vi "TRAJECTORY_CREATE_CUBIC_BEGIN.vi"() -> (0 "Trajectory \ncalculation \nerror":errorcluster, 2 "Trajectory Items":i32, 3 "TotalTImeSecs":dbl)   [LabVIEW 2019]
uses:
  <vilib>/Rock Robotics/WPI/ThirdParty/JAS_Junk/TrajLib/Rotation_CreateAngle.vi
  <vilib>/Rock Robotics/WPI/ThirdParty/JAS_Junk/TrajLib/DiffDriveKinematicsConstraint_New.vi
  <vilib>/Rock Robotics/WPI/ThirdParty/JAS_Junk/TrajLib/CentripetalAccelConstraint_New.vi
  <vilib>/Rock Robotics/WPI/ThirdParty/JAS_Junk/TrajLib/Trajectory_Library.lvlib
panel:
  in  "Interior WayPoints":cluster{"X Inches":dbl, "Y Inches":dbl}[](array[cluster])=[{"X Inches"=105.0, "Y Inches"=65.0}]
  in  "Output Position":T1={"X Inches"=210.0, "Y Inches"=106.0, "Heading\nDegrees"=45.0}
  in  "Input Position":T1={"X Inches"=15.0, "Y Inches"=105.0, "Heading\nDegrees"=-45.0}
  in  "Use Diff Drive\nKinematic\nConstraint":bool=TRUE
  in  "Use Centripetal\nAcceleration\nConstaint":bool=TRUE
  out "Wheelbase Width":dbl=0.66 format="%20.4f"
  out "MaxAcceleration":dbl=1.3 format="%17.4f"
  out "MaxVelocity":dbl=2.0 format="%17.4f"
  out "Max Cent Accel":dbl=1.0 format="%20.4f"
  in  "Max Cent Accel INCHES/SEC^2":dbl=15.0 format="%20.1f"
  in  "Wheelbase Width INCHES":dbl=50.0 format="%20.1f"
  in  "MaxAcceleration INCHES/SEC^2":dbl=35.0 format="%17.1f"
  in  "MaxVelocity  INCHES/SEC":dbl=45.0 format="%17.1f"
  # "TRAJECTORY CONFIGURATION"
  # "real 20.9"
  # "TRAJECTORY DEFINITION"
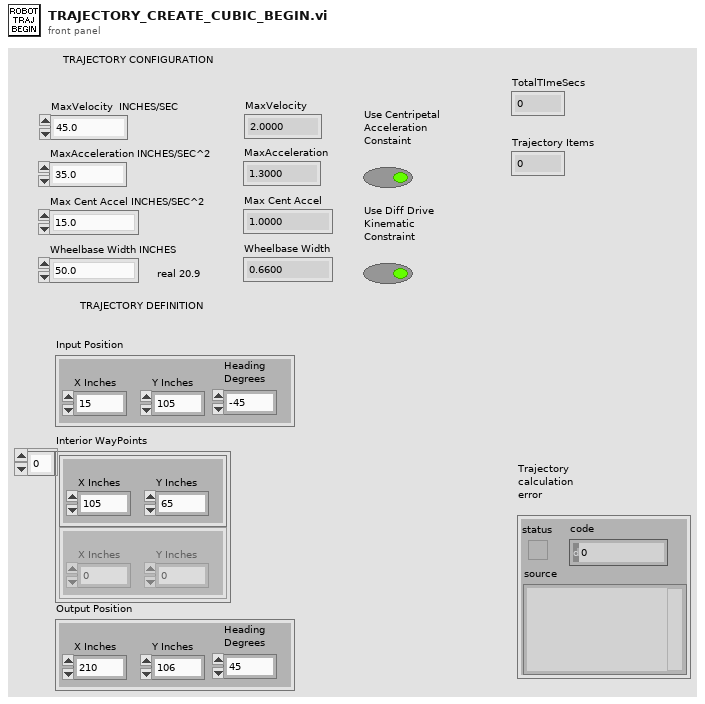
[diagram p1: front panel]
types:
  T1 = cluster{"X Inches":dbl, "Y Inches":dbl, "Heading\nDegrees":dbl}
  T2 = typedef "Trajectory_Library.lvlib/TRANSLATION2D.ctl" = cluster{"X":dbl, "Y":dbl}
  T3 = typedef "Trajectory_Library.lvlib/POSE2D.ctl" = cluster{"TRANSLATION":T2, "ROTATION":T4}
  T4 = typedef "Trajectory_Library.lvlib/ROTATION2D.ctl" = cluster{"VALUE":dbl, "COS":dbl, "SIN":dbl}
  T5 = typedef "Trajectory_Library.lvlib/TRAJ_CONFIG.ctl" = cluster{"MaxVelocity":dbl, "Max Acceleration":dbl, "StartVelocity":dbl, "End Velocity":dbl, "Reversed":bool, "DiffDrKineConstntDefined":bool, "CentAcellConstntDefined":bool, "DiffDrVoltConstntDefined":bool, "DIFF_DRIVE_KINE_CONSTRAINT":T6, "CENTRIPETAL_ACCEL_CONSTRAINT":T8, "SwerveDrKineConstntDefined":bool, "SWERVE_DRIVE_KINE_CONSTRAINT":T9, "DIFF_DRIVE_VOLTAGE_CONSTRAINT":T12, "MECANUM_DRIVE_KINE_CONSTRAINT":T14, "MecanumDrKineConstntDefined":bool}
  T6 = typedef "Trajectory_Library.lvlib/TRAJ_CONSTRAINT_DIIF_DRIVE_KINEMATICS.ctl" = cluster{"Max Speed (M/S)":dbl, "DIFF_DRIVE_KINEMATICS":T7}
  T7 = typedef "Trajectory_Library.lvlib/DIFF_DRIVE_KINEMATICS.ctl" = cluster{"TrackWidth_Meters":dbl}
  T8 = typedef "Trajectory_Library.lvlib/TRAJ_CONSTRAINT_CENTRIPETAL_ACCEL.ctl" = cluster{"Max Cent Accel":dbl}
  T9 = typedef "Trajectory_Library.lvlib/TRAJ_CONSTRAINT_SWERVE_DRIVE_KINEMATICS.ctl" = cluster{"Max Speed (M/S)":dbl, "SwerveKinematics":T10}
  T10 = typedef "Trajectory_Library.lvlib/SWERVE_DRIVE_KINEMATICS.ctl" = cluster{"NumModules":i32, "InverseKinematics":T11, "ForwardKinematics":T11, "Modules":T2[], "PrevCoR":T2}
  T11 = typedef "NI_Matrix.lvlib/RealMatrix.ctl" = dbl[][]
  T12 = typedef "Trajectory_Library.lvlib/TRAJ_CONSTRAINT_DIIF_DRIVE_VOLTAGE.ctl" = cluster{"Max Voltage":dbl, "DIFF_DRIVE_KINEMATICS":T7, "SIMPLE_MOTOR_FF":T13}
  T13 = typedef "Trajectory_Library.lvlib/SIMPLE_MOTOR_FF.ctl" = cluster{"Ks":dbl, "Kv":dbl, "Ka":dbl}
  T14 = typedef "Trajectory_Library.lvlib/TRAJ_CONSTRAINT_MECA_DRIVE_KINEMATICS.ctl" = cluster{"Max Speed (M/S)":dbl, "MECA_DRIVE_KINEMATICS":T15}
  T15 = typedef "Trajectory_Library.lvlib/MECA_DRIVE_KINEMATICS.ctl" = cluster{"FrontLeft":T2, "FrontRight":T2, "RearLeft":T2, "RearRight":T2, "InverseKinematics":T11, "ForwardKinematics":T11, "PrevCoR":T2}
  T16 = typedef "Trajectory_Library.lvlib/TRAJECTORY.ctl" = cluster{"TotalTImeSecs":dbl, "States":T17[]}
  T17 = typedef "Trajectory_Library.lvlib/TRAJ_STATE.ctl" = cluster{"TimeSeconds":dbl, "Velocity":dbl, "Acceleration":dbl, "POSE":T3, "Curvature":dbl}
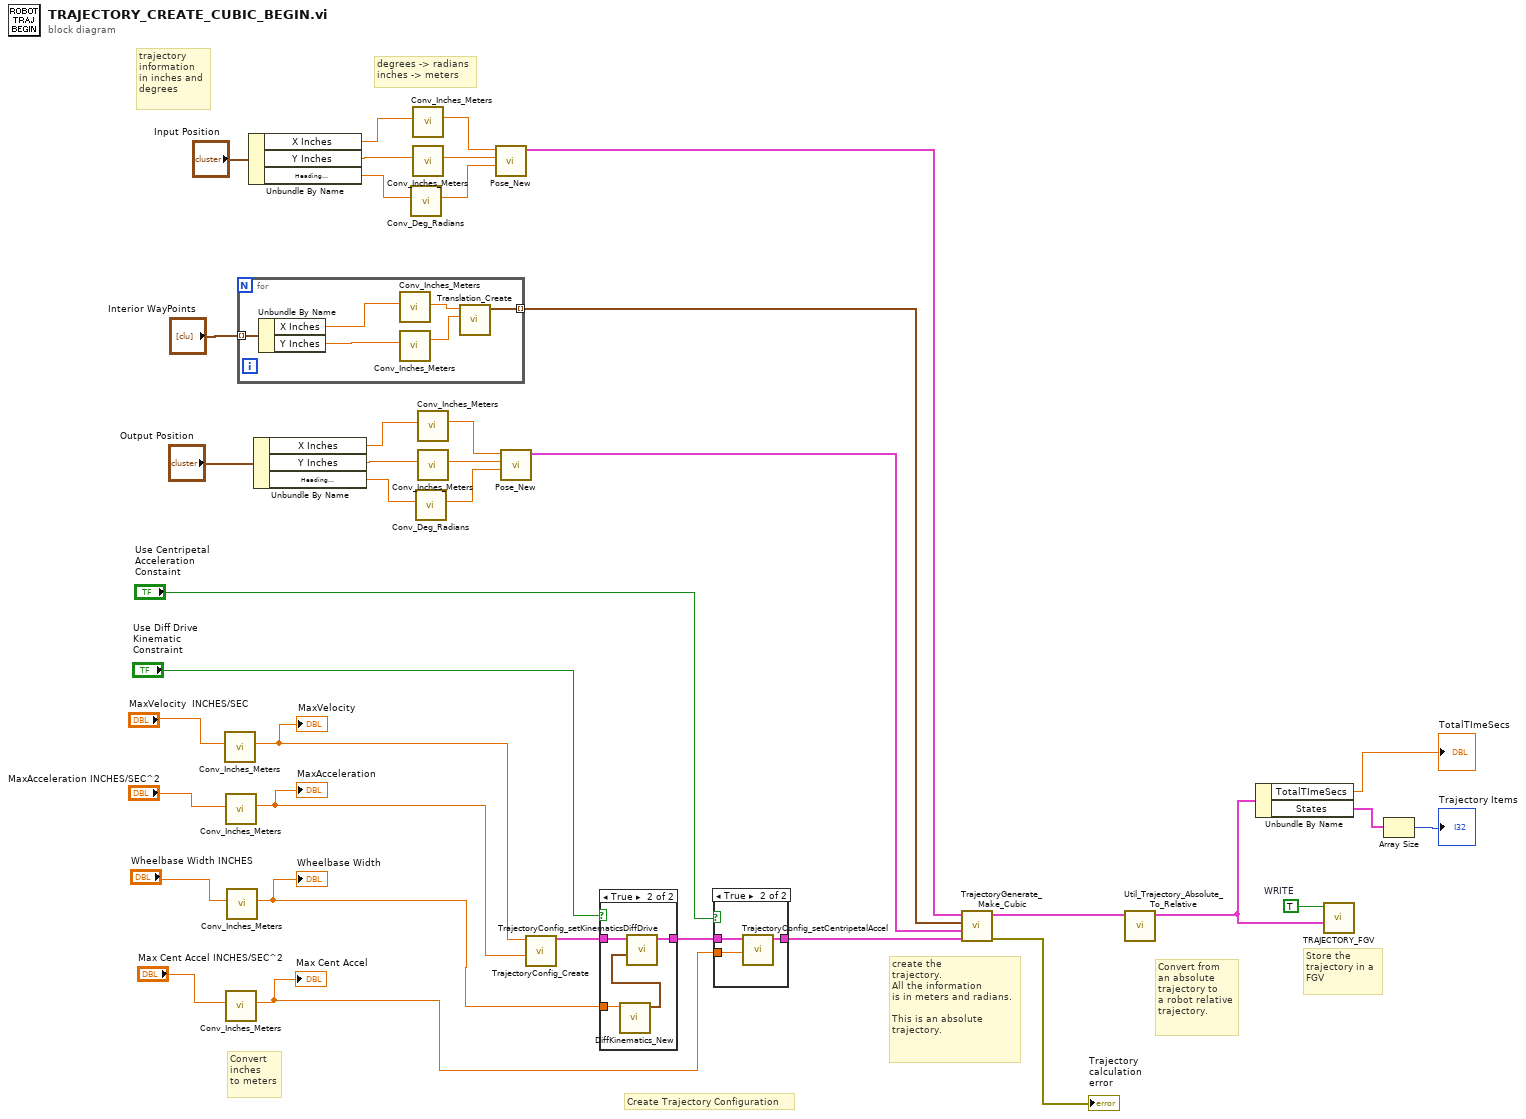
[diagram p0: block diagram]
diagram:
  w6 = TRUE  # WRITE
  # "Store the\ntrajectory in a \nFGV"
  # "Convert from\nan absolute\ntrajectory to\na robot relative\ntrajectory."
  # "Convert\ninches\nto meters"
  # "degrees -> radians\ninches -> meters"
  # "create the\ntrajectory.\nAll the information\nis in meters and radians.\n\nThis is an absolute \ntrajectory."
  # "trajectory\ninformation\nin inches and\ndegrees"
  # "Create Trajectory Configuration"
  n1 = call <vilib>:"Conv_Inches_Meters.vi"("INCH"="MaxVelocity  INCHES/SEC") -> ("Meters"=w27:dbl)  [unwired: 10 in]
  "MaxVelocity" <- w27
  n2 = call <vilib>:"Conv_Inches_Meters.vi"("INCH"="MaxAcceleration INCHES/SEC^2") -> ("Meters"=w28:dbl)  [unwired: 10 in]
  "MaxAcceleration" <- w28
  n3 = call <vilib>:"Conv_Inches_Meters.vi"("INCH"="Max Cent Accel INCHES/SEC^2") -> ("Meters"=w29:dbl)  [unwired: 10 in]
  "Max Cent Accel" <- w29
  n4 = call <vilib>:"Conv_Inches_Meters.vi"("INCH"="Wheelbase Width INCHES") -> ("Meters"=w30:dbl)  [unwired: 10 in]
  "Wheelbase Width" <- w30
  n5 = for {
    tunnel: "Interior WayPoints" -> [w42] mode=indexing
    tunnel: [w39] -> w8 mode=indexing
    n6 = Unbundle By Name(w42) -> ("X Inches"=w44:dbl, "Y Inches"=w43:dbl)
    n7 = call <vilib>:"Conv_Inches_Meters.vi"("INCH"=w44) -> ("Meters"=w41:dbl)  [unwired: 10 in]
    n8 = call <vilib>:"Conv_Inches_Meters.vi"("INCH"=w43) -> ("Meters"=w40:dbl)  [unwired: 10 in]
    n9 = call <vilib>:"Translation_Create.vi"("Y"=w40, "X"=w41) -> ("TRANSLATION"=w39:T2)  [unwired: 9 in]
  }
  n10 = Unbundle By Name("Input Position") -> ("X Inches"=w23:dbl, "Y Inches"=w22:dbl, "Heading\nDegrees"=w20:dbl)
  n11 = Unbundle By Name("Output Position") -> ("X Inches"=w16:dbl, "Y Inches"=w15:dbl, "Heading\nDegrees"=w13:dbl)
  n12 = call <vilib>:"Conv_Deg_Radians.vi"("Degress"=w20) -> ("Radians"=w21:dbl)  [unwired: 10 in]
  n13 = call <vilib>:"Conv_Inches_Meters.vi"("INCH"=w23) -> ("Meters"=w18:dbl)  [unwired: 10 in]
  n14 = call <vilib>:"Conv_Inches_Meters.vi"("INCH"=w22) -> ("Meters"=w19:dbl)  [unwired: 10 in]
  n15 = call <vilib>:"Conv_Deg_Radians.vi"("Degress"=w13) -> ("Radians"=w14:dbl)  [unwired: 10 in]
  n16 = call <vilib>:"Conv_Inches_Meters.vi"("INCH"=w16) -> ("Meters"=w11:dbl)  [unwired: 10 in]
  n17 = call <vilib>:"Conv_Inches_Meters.vi"("INCH"=w15) -> ("Meters"=w12:dbl)  [unwired: 10 in]
  n18 = call <vilib>:"Pose_New.vi"("Heading"=w21, "Y"=w19, "X"=w18) -> ("out POSe"=w7:T3)  [unwired: 8 in]
  n19 = call <vilib>:"Pose_New.vi"("Heading"=w14, "Y"=w12, "X"=w11) -> ("out POSe"=w9:T3)  [unwired: 8 in]
  n20 = call <vilib>:"TrajectoryConfig_Create.vi"("MaxAcceleration"=w28, "MaxVelocity"=w27) -> ("TRAJECTORY_CONFIG"=w34:T5)  [unwired: 9 in]
  n21 = case shown="True" "Use Diff Drive\nKinematic\nConstraint" {
    tunnel: w34 -> [w45 w49]
    tunnel: [w45 w48] -> w33
    tunnel: w30 -> [_ w46]
    frame False {
    }
    frame True {
      n22 = call <vilib>:"DiffKinematics_New.vi"("TrackWidth_Meters"=w46) -> ("DIFF_DRIVE_KINEMATICS"=w47:T7)  [unwired: 10 in]
      n23 = call <vilib>:"TrajectoryConfig_setKinematicsDiffDrive.vi"("DIFF_DRIVE_KINEMATICS"=w47, "inTRAJECTORY_CONFIG"=w49) -> ("outTRAJECTORY_CONFIG"=w48:T5)  [unwired: 9 in]
    }
  }
  n24 = case shown="True" "Use Centripetal\nAcceleration\nConstaint" {
    tunnel: w33 -> [w50 w53]
    tunnel: [w50 w52] -> w25
    tunnel: w29 -> [_ w51]
    frame False {
    }
    frame True {
      n25 = call <vilib>:"TrajectoryConfig_setCentripetalAccel.vi"("Max Cent Accel"=w51, "inTRAJECTORY_CONFIG"=w53) -> ("outTRAJECTORY_CONFIG"=w52:T5)  [unwired: 9 in]
    }
  }
  n26 = call <vilib>:"TrajectoryGenerate_Make_Cubic.vi"("traj_config"=w25, "Enging POSE"=w9, "Interior WAYPOINTS"=w8, "Starting POSE"=w7) -> ("error out"=→"Trajectory \ncalculation \nerror":errorcluster, "TRAJECTORY"=w1:T16)  [unwired: 6 in]
  n27 = call <vilib>:"Util_Trajectory_Absolute_To_Relative.vi"("absTRAJECTORY"=w1) -> ("outputRelativeTRAJECTORY"=w2:T16)  [unwired: 10 in]
  n28 = Unbundle By Name(w2) -> ("TotalTImeSecs"=→"TotalTImeSecs":dbl, "States"=w4:T17[])
  n29 = call "TRAJECTORY_FGV.vi"("inTRAJECTORY"=w2, "WRITE"=w6) -> ()  [unwired: 9 in, 1 out]
  n30 = Array Size(array=w4) -> (size(s)=→"Trajectory Items":i32)
